vi "Inverse A x Y using SVD (DBL).vi"(8 "Known Vector":dbl[](array[numeric]), 9 "V":T1, 10 "1/S":dbl[](array[numeric]), 11 "U*":T1) -> (0 "error":i32, 3 "Solution Vector":dbl[](array[numeric]))   [LabVIEW 2014, in "NI_AALPro.lvlib"]
uses:
  NI_AALPro.lvlib
  RealMatrix.ctl
  A x Vector.vi
  NI_AALBase.lvlib
  NI_Matrix.lvlib
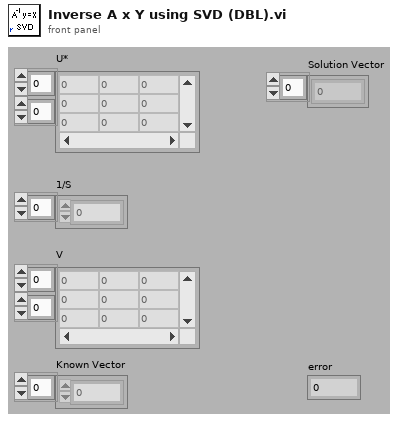
[diagram p1: front panel]
types:
  T1 = typedef "NI_Matrix.lvlib/RealMatrix.ctl" = dbl[][]
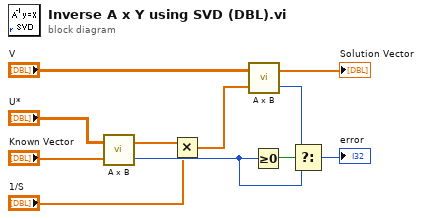
[diagram p0: block diagram]
diagram:
  n1 = call-poly "A x B.vi"("Vector"="Known Vector", "A"="U*") -> ("error"=w5:i32, "A x Vector"=w3:dbl[])
  n2 = Multiply(x=w3, y="1/S") -> (x*y=w1:dbl[])
  n3 = call-poly "A x B.vi"("Vector"=w1, "A"="V") -> ("error"=w6:i32, "A x Vector"=→"Solution Vector":dbl[])
  n4 = Greater Or Equal To 0?(x=w5) -> (x >= 0?=w7:bool)
  n5 = Select(t=w6, s=w7, f=w5) -> (s? t:f=→"error":i32)
